vi "Parse Data Type.vi"(10 "Numeric(1)":u8) -> (2 "Data Type":T1)   [LabVIEW 2014, in "hse-db.lvlib" / "MySQL (TCP).lvlib"]
uses:
  MySQL (TCP).lvlib
  Controls/Data Types.ctl
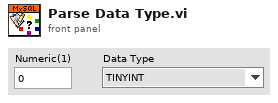
[diagram p1: front panel]
types:
  T1 = typedef "hse-db.lvlib/MySQL (TCP).lvlib/Data Types.ctl" = enum16{"TINYINT", "SMALLINT", "MEDIUMINT", "INT", "BIGINT", "FLOAT", "DOUBLE", "NULL", "DECIMAL", "BIT", "CHAR", "VARCHAR", "TINYTEXT", "TEXT", "MEDIUMTEXT", "LONGTEXT", "BINARY", "VARBINARY", "TINYBLOB", "BLOB", "MEDIUMBLOB", "LONGBLOB", "ENUM", "SET", "DATE", "DATETIME", "TIME", "TIMESTAMP", "YEAR", "GEOMETRY"}
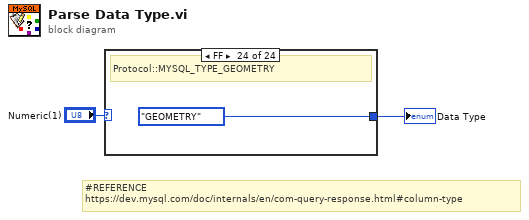
[diagram p0: block diagram]
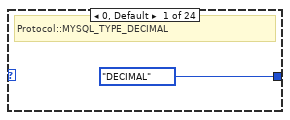
[diagram p2: hidden frame]
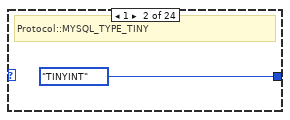
[diagram p3: hidden frame]
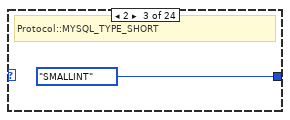
[diagram p4: hidden frame]
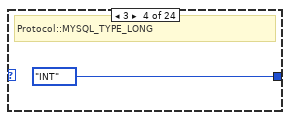
[diagram p5: hidden frame]
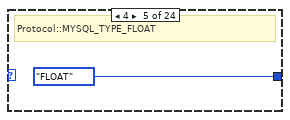
[diagram p6: hidden frame]
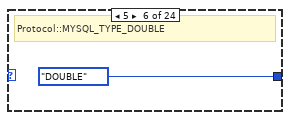
[diagram p7: hidden frame]
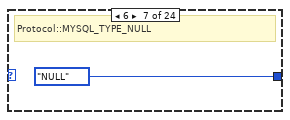
[diagram p8: hidden frame]
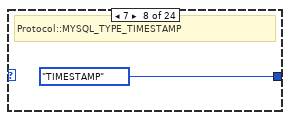
[diagram p9: hidden frame]
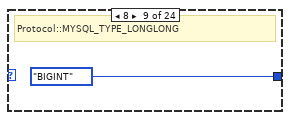
[diagram p10: hidden frame]
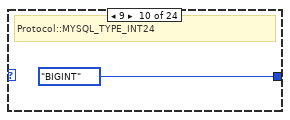
[diagram p11: hidden frame]
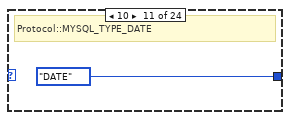
[diagram p12: hidden frame]
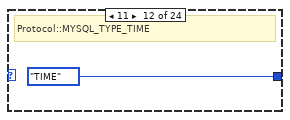
[diagram p13: hidden frame]
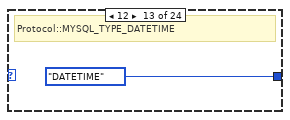
[diagram p14: hidden frame]
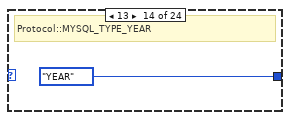
[diagram p15: hidden frame]
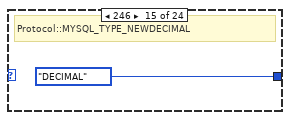
[diagram p16: hidden frame]
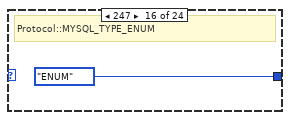
[diagram p17: hidden frame]
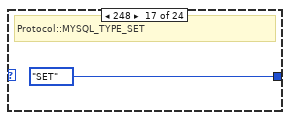
[diagram p18: hidden frame]
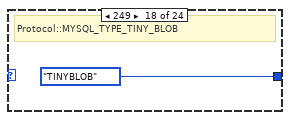
[diagram p19: hidden frame]
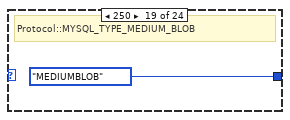
[diagram p20: hidden frame]
diagram:
  # "#REFERENCE\nhttps://dev.mysql.com/doc/internals/en/com-query-response.html#column-type"
  n1 = case shown="FF" "Numeric(1)" {
    tunnel: [Data_Types."DECIMAL" ("MySQLDataTypes") Data_Types."TINYINT" ("MySQLDataTypes") Data_Types."SMALLINT" ("MySQLDataTypes") Data_Types."INT" ("MySQLDataTypes") Data_Types."FLOAT" ("MySQLDataTypes") Data_Types."DOUBLE" ("MySQLDataTypes") Data_Types."NULL" ("MySQLDataTypes") Data_Types."TIMESTAMP" ("MySQLDataTypes") Data_Types."BIGINT" ("MySQLDataTypes") Data_Types."BIGINT" ("MySQLDataTypes") Data_Types."DATE" ("MySQLDataTypes") Data_Types."TIME" ("MySQLDataTypes") Data_Types."DATETIME" ("MySQLDataTypes") Data_Types."YEAR" ("MySQLDataTypes") Data_Types."DECIMAL" ("MySQLDataTypes") Data_Types."ENUM" ("MySQLDataTypes") Data_Types."SET" ("MySQLDataTypes") Data_Types."TINYBLOB" ("MySQLDataTypes") Data_Types."MEDIUMBLOB" ("MySQLDataTypes") Data_Types."LONGBLOB" ("MySQLDataTypes") Data_Types."BLOB" ("MySQLDataTypes") Data_Types."VARCHAR" ("MySQLDataTypes") Data_Types."TEXT" ("MySQLDataTypes") Data_Types."GEOMETRY" ("MySQLDataTypes")] -> w1
    frame 0, Default {
      # "Protocol::MYSQL_TYPE_DECIMAL"
    }
    frame 1 {
      # "Protocol::MYSQL_TYPE_TINY"
    }
    frame 2 {
      # "Protocol::MYSQL_TYPE_SHORT"
    }
    frame 3 {
      # "Protocol::MYSQL_TYPE_LONG"
    }
    frame 4 {
      # "Protocol::MYSQL_TYPE_FLOAT"
    }
    frame 5 {
      # "Protocol::MYSQL_TYPE_DOUBLE"
    }
    frame 6 {
      # "Protocol::MYSQL_TYPE_NULL"
    }
    frame 7 {
      # "Protocol::MYSQL_TYPE_TIMESTAMP"
    }
    frame 8 {
      # "Protocol::MYSQL_TYPE_LONGLONG"
    }
    frame 9 {
      # "Protocol::MYSQL_TYPE_INT24"
    }
    frame 10 {
      # "Protocol::MYSQL_TYPE_DATE"
    }
    frame 11 {
      # "Protocol::MYSQL_TYPE_TIME"
    }
    frame 12 {
      # "Protocol::MYSQL_TYPE_DATETIME"
    }
    frame 13 {
      # "Protocol::MYSQL_TYPE_YEAR"
    }
    frame 246 {
      # "Protocol::MYSQL_TYPE_NEWDECIMAL"
    }
    frame 247 {
      # "Protocol::MYSQL_TYPE_ENUM"
    }
    frame 248 {
      # "Protocol::MYSQL_TYPE_SET"
    }
    frame 249 {
      # "Protocol::MYSQL_TYPE_TINY_BLOB"
    }
    frame 250 {
      # "Protocol::MYSQL_TYPE_MEDIUM_BLOB"
    }
    frame 251 {
      # "Protocol::MYSQL_TYPE_LONG_BLOB"
    }
    frame 252 {
      # "Protocol::MYSQL_TYPE_BLOB"
    }
    frame 253 {
      # "Protocol::MYSQL_TYPE_VAR_STRING"
    }
    frame 254 {
      # "Protocol::MYSQL_TYPE_STRING"
    }
    frame 255 {
      # "Protocol::MYSQL_TYPE_GEOMETRY"
    }
  }
  "Data Type" <- w1
